vi "Beat_v2.vi"(7 "Name (\"\" to Use UUID)":string="Beat") -> ()   [LabVIEW 2025]
doc: "Compact code template for creating a CSM module without a user interface. The functionality of this template is identical to the CSM Module Template VI.\n\n\n> [!NOTE] <b>CSM Naming Rules</b>\n>\n> - CSM module name must be unique. Otherwise, CSM enters a `Critical Error` state.\n> - If the input module name is an empty string (\"\"), the system uses a UUID as the module name. Such a module is marked as standalone mode and does not appear in the module list.\n> - Worker Mode Rule: If the input module name ends with `#`, a worker mode node will be instantiated. Multiple worker mode nodes can form a worker mode module.\n> - Chain of Responsibility Mode Rule: If the input module name ends with `$` followed by a number, a chain of responsibility mode node will be instantiated. Multiple chain of responsibility mode nodes can form a chain of responsibility mode module.\n> - System-Level Module Rule: If the input module name starts with `.`, the module is a system-level module. Under default settings, such modules are not listed by the CSM - List Modules VI and are suitable for instantiating modules that run in the background.\n> - Submodule Rule: `.` is also allowed in a module name to separate the module name into multiple parts. CSM does not have strict rules for submodules. The `.` in the module name only marks the logical relationship between different modules. From an execution perspective, they are considered independent modules. The only difference is that you can obtain a list of logical submodules via the CSM - List Submodules VI.\n\n\n-- <b>Controls</b> --\n- <b>Name (\"\" to use UUID)</b>: CSM module name. Refer to <b>CSM Naming Rules</b> for module naming rules."
uses:
  <userlib>/_NEVSTOP/Communicable State Machine(CSM)/AdvanceAPI/CSM - Revert Arguments-Safe String.vi
  <userlib>/_NEVSTOP/Communicable State Machine(CSM)/_Shared/Trim Single-line Text.vi
  <userlib>/_NEVSTOP/Communicable State Machine(CSM)/AdvanceAPI/CSM - Break Down Multiple States String.vi
  <userlib>/_NEVSTOP/Communicable State Machine(CSM)/AdvanceAPI/CSM - Compact Multiple States.vi
  <userlib>/_NEVSTOP/Communicable State Machine(CSM)/AdvanceAPI/CSM - Make String Arguments Safe.vi
  <userlib>/_NEVSTOP/Communicable State Machine(CSM)/AdvanceAPI/CSM - Keywords.vi
  <userlib>/_NEVSTOP/Communicable State Machine(CSM)/Communicable State Machine.lvlib
panel:
  in  "Array 2":i32[](array[numeric])
  out "BeatInterval":i32
  out "State History":string
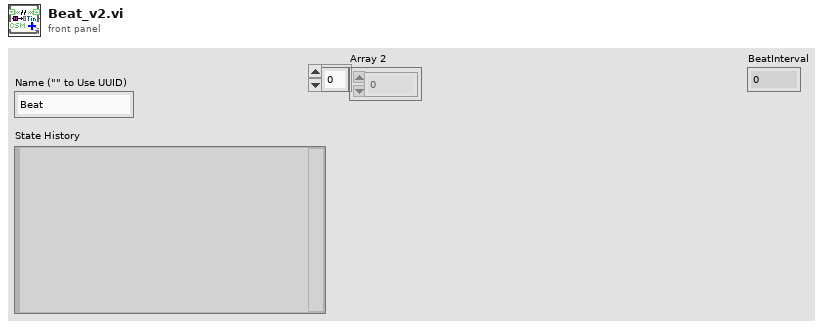
[diagram p1: front panel]
types:
  T1 = enum32{"Invalid", "Standard", "Closed", "Hidden", "Minimized", "Maximized"}
  T2 = enum32{"invalid app kind", "Development System", "Run Time System", "Student Edition", "Embedded LabVIEW", "Evaluation", "Custom"}
  T3 = typedef "Communicable State Machine.lvlib/_CSM_Response Source Message.ctl" = cluster{"‘State":string, "’Arguments":string, "’Error":errorcluster}
  T4 = cluster{"Current VI Reference":refnum<vi>, "Close Panel on Exit?":bool}
  T5 = cluster{"Core":cluster{"Current VI Reference":refnum<vi>, "Close Panel on Exit?":bool}, "BeatActive":bool, "T0":i32, "BeatInterval":i32, "N":i32}
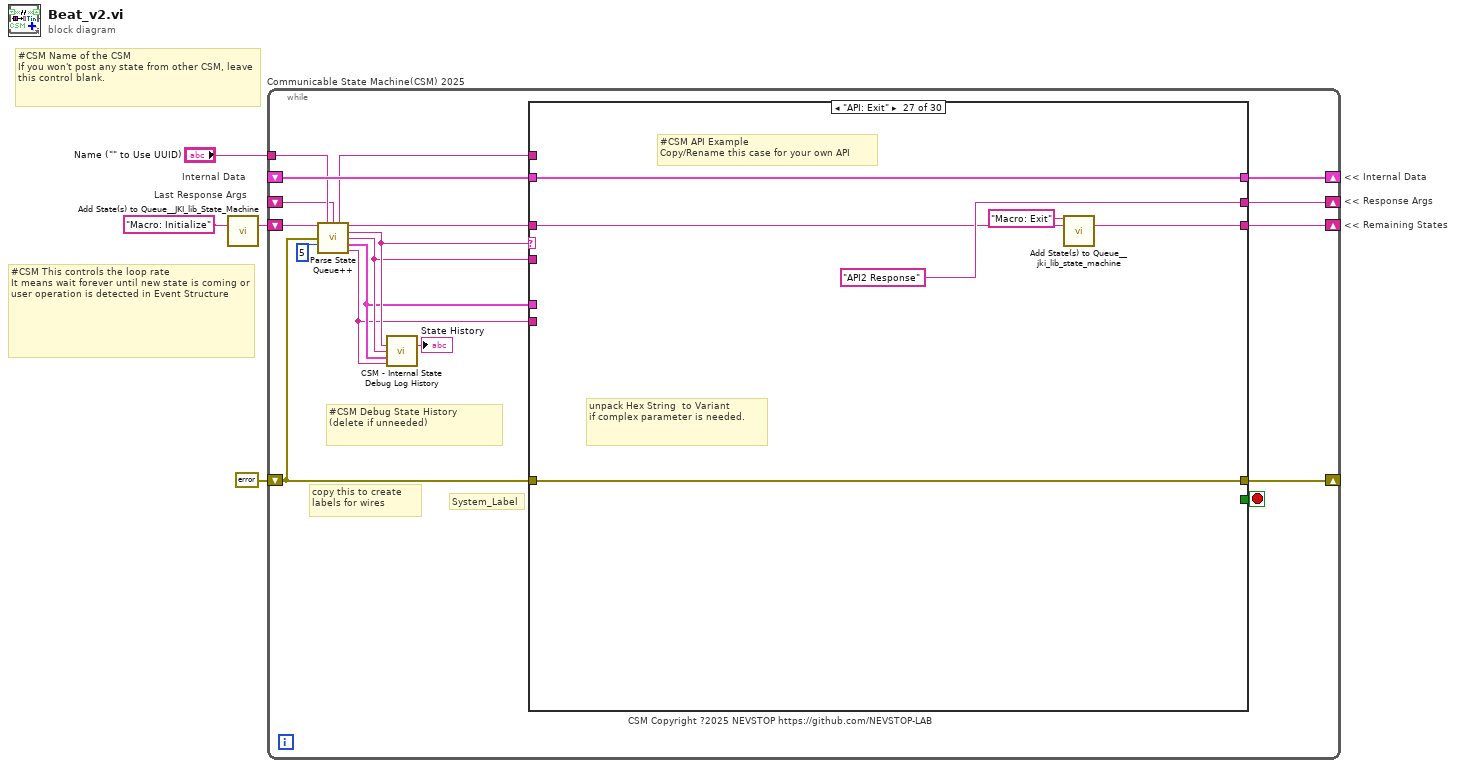
[diagram p0: block diagram]
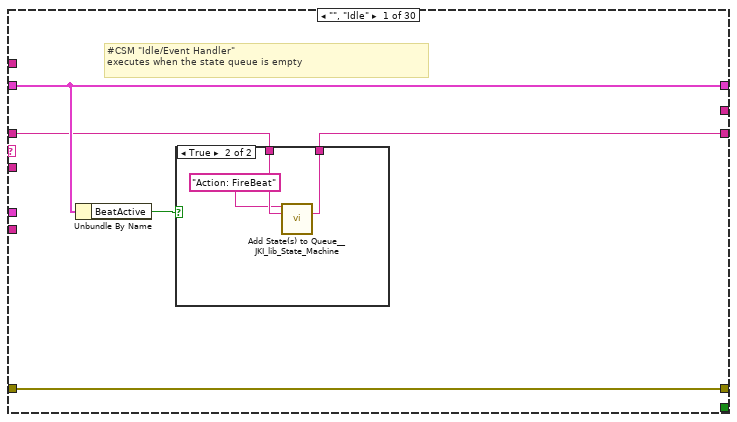
[diagram p2: hidden frame]
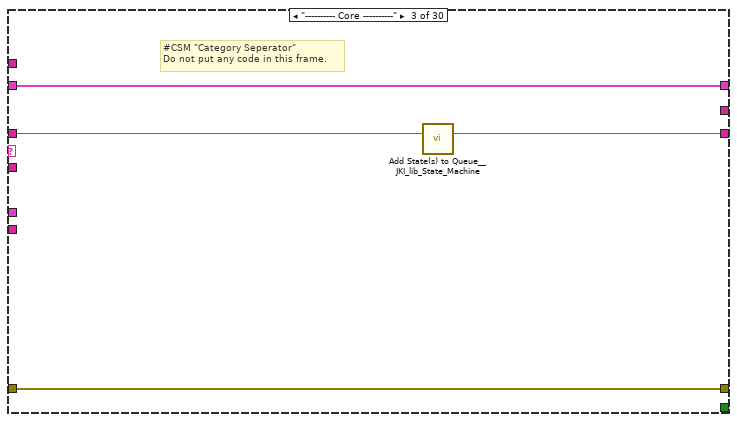
[diagram p5: hidden frame]
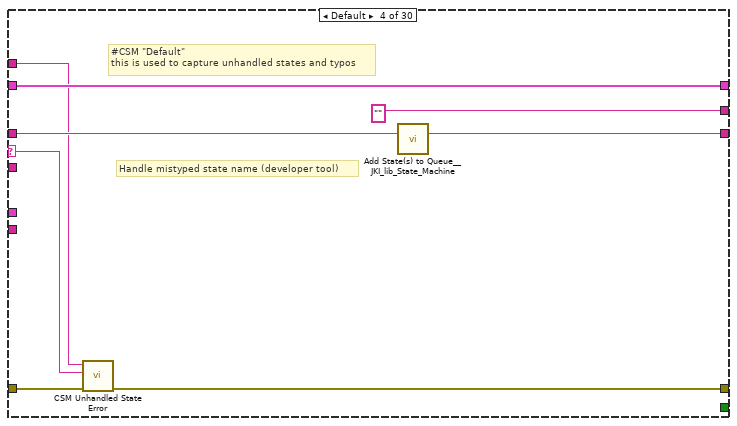
[diagram p6: hidden frame]
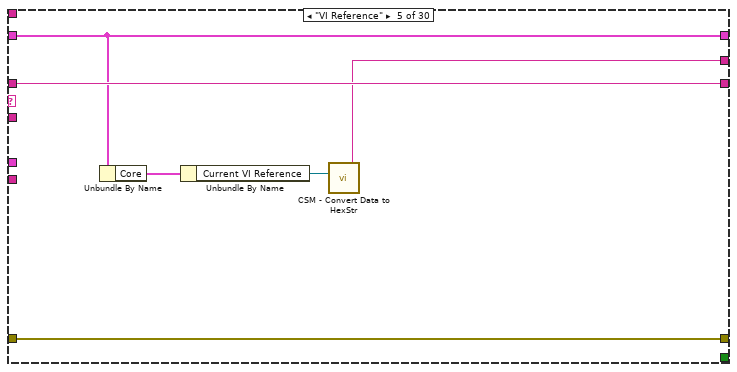
[diagram p7: hidden frame]
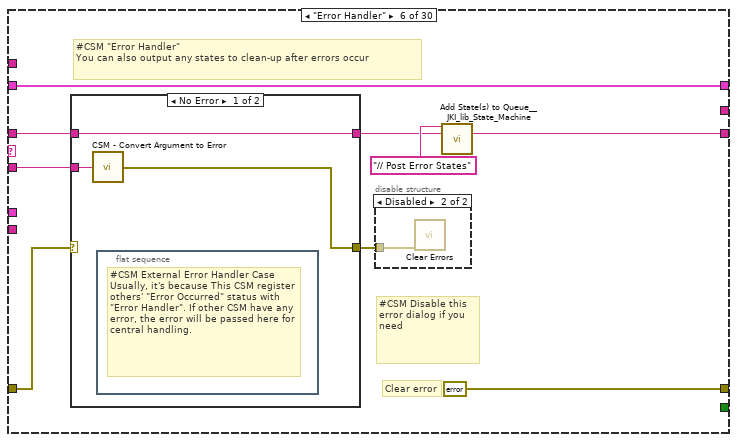
[diagram p8: hidden frame]
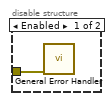
[diagram p9: hidden frame]
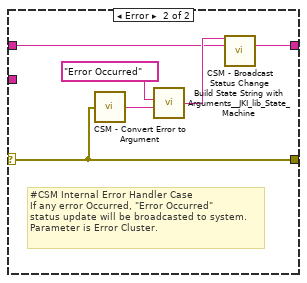
[diagram p10: hidden frame]
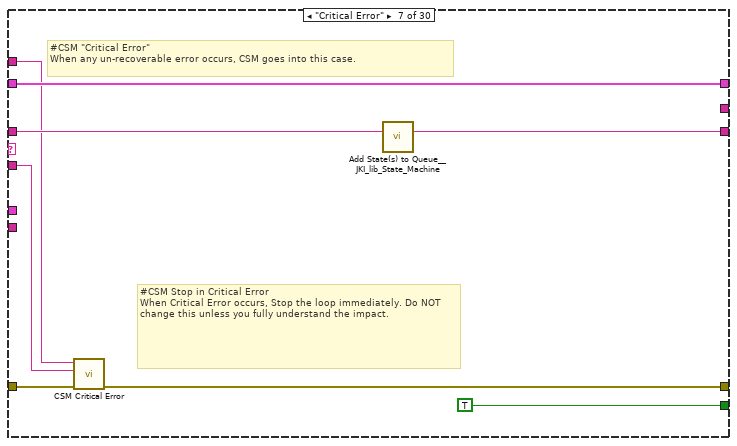
[diagram p11: hidden frame]
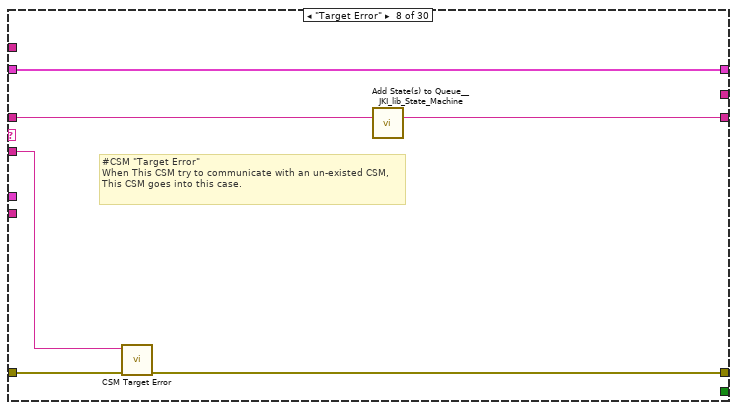
[diagram p12: hidden frame]
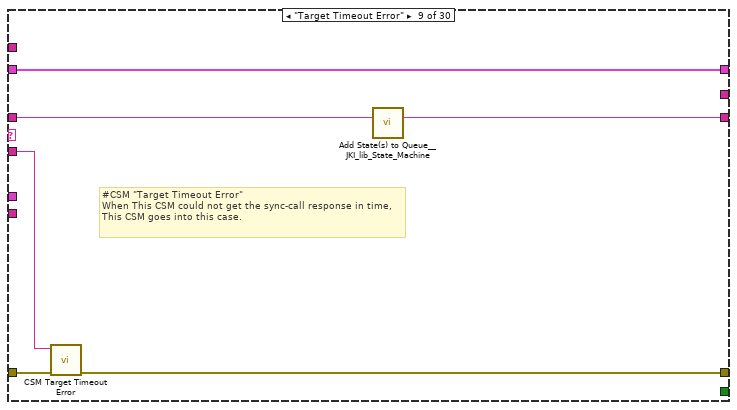
[diagram p13: hidden frame]
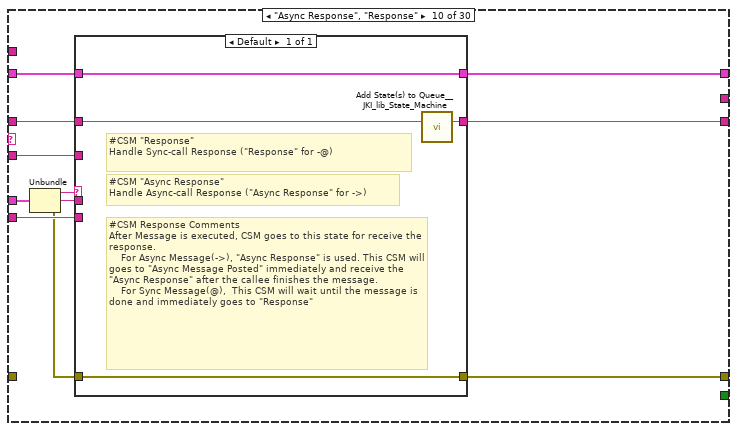
[diagram p14: hidden frame]
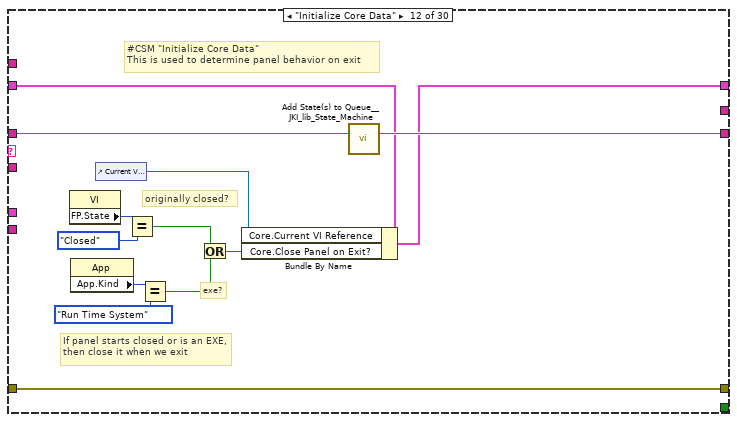
[diagram p16: hidden frame]
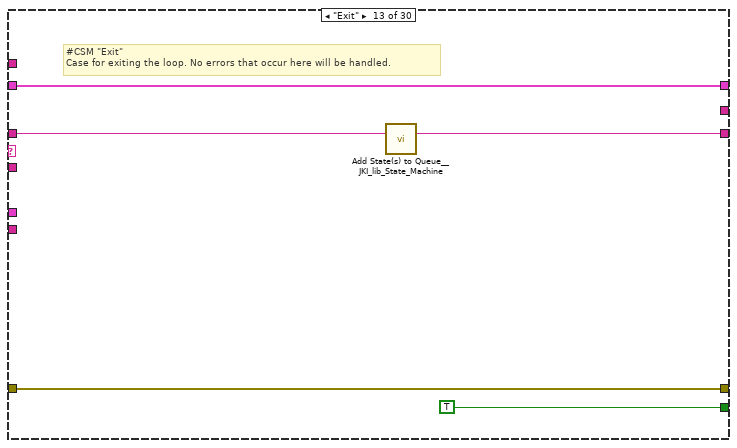
[diagram p17: hidden frame]
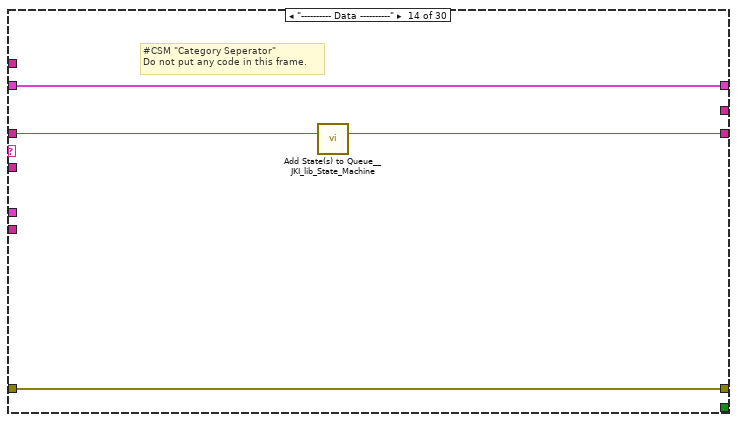
[diagram p18: hidden frame]
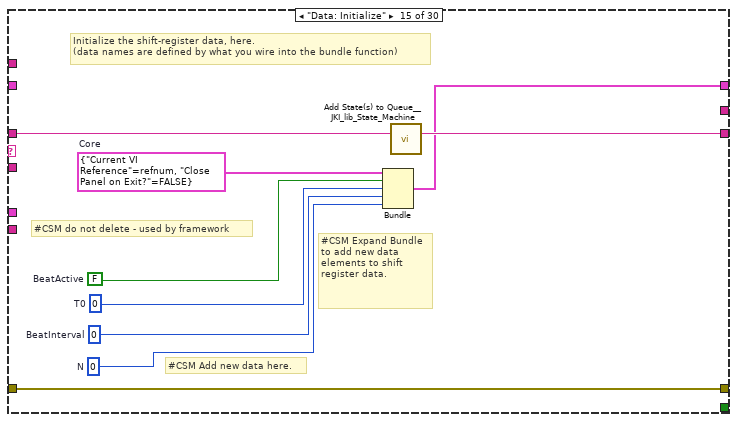
[diagram p19: hidden frame]
diagram:
  # "Last Response Args"
  # "Internal Data"
  # "#CSM Name of the CSM\nIf you won't post any state from other CSM, leave this control blank."
  # "#CSM This controls the loop rate\nIt means wait forever until new state is coming or user operation is detected in Event Structure"
  # "<< Internal Data"
  # "<< Response Args"
  # "<< Remaining States"
  n1 = call <vilib>:"Add State(s) to Queue__JKI_lib_State_Machine.vi"("State(s) in (\"\")"="Macro: Initialize" ("Init State(\"Macro: Initialize\")")) -> ("States Out"=w4:string)  [unwired: 14 in]
  n2 = while "Communicable State Machine(CSM) 2025" {
    shift-right: [w17] -> _
    shift-left: _ -> [w16]
    shift-right: [w20] -> _
    shift-left: errorcluster {"status"=FALSE, "code"=0, "source"=""} ("error out") -> [w15]
    shift-right: [w19] -> _
    shift-left: w4 -> [w21]
    tunnel: "Name (\"\" to Use UUID)" -> [w13]
    shift-right: [w14] -> _
    shift-left: _ -> [w7]
    stop <- w18 stop-if-true
    # "#CSM Debug State History\n(delete if unneeded)"
    # "copy this to create labels for wires"
    # "System_Label"
    # "CSM Copyright ?2025 NEVSTOP https://github.com/NEVSTOP-LAB"
    n3 = call <userlib>:"Parse State Queue++.vi"("State Queue"=w21, "Name (\"\" to Use UUID)"=w13, "Response Arguments"=w7, "Previous Error"=w15, "Dequeue (1 ms)"=5 ("Timeout")) -> ("Name Used"=w8:string, "Remaining States"=w22:string, "Current State"=w12:string, "Arguments"=w11:string, "Additional Information"=w10:T3, "Source CSM"=w9:string)  [unwired: 5 in]
    n4 = call <userlib>:"CSM - Internal State Debug Log History.vi"("State"=w12, "Arguments (\"\")"=w11, ">> Response Source Message >>"=w10, "Source (\"\")"=w9) -> ("Debug Log"=→"State History":string)  [unwired: 11 in]
    n5 = case shown="\"API: Exit\"" w12 {
      selector: w12 -> [_ _ _ w41 _ _ _ _ _ _ _ _ _ _ _ _ _ _ _ _ _ _ _ _ _ _ _ _ _ _]
      tunnel: w22 -> [w24 w33 w38 w45 w51 w57 w78 w84 w90 w98 w109 w123 w128 w132 w141 w143 w150 w154 w158 w164 w179 w248 w253 w260 w262 w266 w283 w291 w305 w321]
      tunnel: w11 -> [_ _ _ _ _ w56 w74 w83 w88 w97 _ _ _ _ _ _ _ _ _ w159 w173 _ _ _ _ w270 _ _ _ _]
      tunnel: w16 -> [w26 w32 w35 w43 w50 w60 w79 w85 w91 w100 w108 w116 w126 w129 _ w142 w145 w151 w156 w162 w175 w245 w250 w257 w261 w269 w286 w288 w292 w317]
      tunnel: [w27 w34 w36 w39 w52 errorcluster {"status"=FALSE, "code"=0, "source"=""} ("error out") w75 w81 w87 w103 w110 w120 w125 w130 w138 w144 w146 w152 w155 w160 w176 w246 w251 w258 w263 w281 w287 w289 w303 w319] -> w20
      tunnel: w15 -> [w27 w34 w36 w46 w52 w58 w80 w82 w89 _ w110 w120 w125 w130 w138 w144 w147 w152 w155 w161 w177 w246 w251 w258 w263 w281 w287 w289 w303 w319]
      tunnel: [w23 w33 w37 w44 w51 w53 w77 w86 w92 w99 w109 w122 w127 w131 w140 w143 w149 w153 w157 w163 w178 w247 w252 w259 w262 w267 w284 w290 w304 w320] -> w19
      tunnel: [_ _ _ _ _ _ TRUE _ _ _ _ _ TRUE _ _ _ _ _ _ _ _ _ _ _ _ _ _ _ _ _] -> w18
      tunnel: [w26 w32 w35 w43 w50 w60 w79 w85 w91 w101 w108 w121 w126 w129 w139 w142 w145 w151 w156 w162 w175 w245 w250 w257 w261 w268 w286 w288 w293 w318] -> w17
      tunnel: w9 -> [_ _ _ _ _ _ _ _ _ w95 _ _ _ _ _ _ _ _ _ _ _ _ _ _ _ _ _ _ _ _]
      tunnel: w10 -> [_ _ _ _ _ _ _ _ _ w102 _ _ _ _ _ _ _ _ _ _ _ _ _ _ _ _ _ _ _ _]
      tunnel: [_ _ _ "" w47 _ _ _ _ _ _ _ _ _ _ _ _ _ _ _ _ _ _ _ _ "API1 Response" "API2 Response" _ _ _] -> w14
      tunnel: w8 -> [_ _ _ w40 _ _ w73 _ _ _ _ _ _ _ _ _ _ _ _ _ _ _ _ _ _ _ _ _ _ _]
      frame "", "Idle" {
        # "#CSM \"Idle/Event Handler\"\nexecutes when the state queue is empty"
        n6 = Unbundle By Name(w26) -> ("BeatActive"=w25:bool)
        n7 = case shown="True" w25 {
          tunnel: w24 -> [w28 w31]
          tunnel: [w28 w30] -> w23
          frame False {
          }
          frame True {
            n8 = call <vilib>:"Add State(s) to Queue__JKI_lib_State_Machine.vi"("State(s) in Front (\"\")"="Action: FireBeat" ("State(s) in Front (\"\")"), "State(s) in (\"\")"=w31) -> ("States Out"=w30:string)  [unwired: 13 in]
          }
        }
      }
      frame "CSM Documentation" {
        # "#CSM README FIRST\n\nCommunicable State Machine(CSM) is a LabVIEW application framework that builds upon JKI State Machine(JKISM). It follows the pattern of JKISM and extends the keywords to describe message communication between modules, including concepts such as Sync-Message, Async-Message, Subscription/Unsubscription of status - essential elements for creating reusable code modules. For more information, please visit the CSM wiki: https://nevstop-lab.github.io/CSM-Wiki/\n\nFor instructions on JKI State Machine, visit: http://jki.net/state-machine/\nFor information about CSM, visit: https://github.com/NEVSTOP-LAB"
        # "#CSM \"Documentation\"\nCase for holding CSM Documenation"
      }
      frame "---------- Core ----------" {
        # "#CSM \"Category Seperator\"\nDo not put any code in this frame."
        n9 = call <vilib>:"Add State(s) to Queue__JKI_lib_State_Machine.vi"("State(s) in (\"\")"=w38) -> ("States Out"=w37:string)  [unwired: 14 in]
      }
      frame Default {
        # "#CSM \"Default\"\nthis is used to capture unhandled states and typos"
        # "Handle mistyped state name (developer tool)"
        n10 = call <userlib>:"CSM Unhandled State Error.vi"("error in (no error)"=w46, "Undefined State"=w41, "CSM Name"=w40) -> ("error out"=w39:errorcluster)  [unwired: 8 in]
        n11 = call <vilib>:"Add State(s) to Queue__JKI_lib_State_Machine.vi"("State(s) in (\"\")"=w45) -> ("States Out"=w44:string)  [unwired: 14 in]
      }
      frame "VI Reference" {
        n12 = Unbundle By Name(w50) -> ("Core"=w49:T4)
        n13 = Unbundle By Name(w49) -> ("Current VI Reference"=w48:refnum<vi>)
        n14 = call <userlib>:"CSM - Convert Data to HexStr.vi"("Variant"=w48) -> ("HEX String (0-9,A-F)"=w47:string)  [unwired: 8 in]
      }
      frame "Error Handler" {
        # "#CSM Disable this error dialog if you need"
        # "#CSM \"Error Handler\"\nYou can also output any states to clean-up after errors occur"
        # "Clear error"
        n15 = case shown="No Error" w58 {
          selector: w58 -> [_ w67]
          tunnel: [w66 w69] -> w54
          tunnel: w57 -> [w66 w68]
          tunnel: w56 -> [w65 _]
          tunnel: [w64 w67] -> w59
          frame No Error {
            n16 = call <userlib>:"CSM - Convert Argument to Error.vi"("Argument"=w65) -> ("Error"=w64:errorcluster)  [unwired: 4 in]
            n17 = flat-sequence {
              frame #0 {
                # "#CSM External Error Handler Case\nUsually, it's because This CSM register others' \"Error Occurred\" status with \"Error Handler\". If other CSM have any error, the error will be passed here for central handling."
              }
            }
          }
          frame Error {
            # "#CSM Internal Error Handler Case \nIf any error Occurred, \"Error Occurred\" \nstatus update will be broadcasted to system.\nParameter is Error Cluster."
            n18 = call <userlib>:"CSM - Convert Error to Argument.vi"("Error"=w67) -> ("Argument"=w71:string)  [unwired: 4 in]
            n19 = call <vilib>:"Build State String with Arguments__JKI_lib_State_Machine.vi"("Arguments (\"\")"=w71, "State"="Error Occurred" ("Status with Arguments")) -> ("State with Arguments"=w70:string)  [unwired: 4 in]
            n20 = call <userlib>:"CSM - Broadcast Status Change.vi"("Status With Arguments"=w70, "State Queue"=w68) -> ("Remaining States"=w69:string)  [unwired: 13 in]
          }
        }
        n21 = disable-structure shown="Disabled" {
          disable-tunnel: w59 -> [w62 w63]
          frame Enabled {
            n22 = call <vilib>:"General Error Handler.vi"("error in (no error)"=w62) -> ()  [unwired: 10 in, 5 out]
          }
          frame Disabled {
            n23 = call <vilib>:"Clear Errors.vi"("error in (no error)"=w63) -> ()  [unwired: 5 in, 2 out]
          }
        }
        n24 = call <vilib>:"Add State(s) to Queue__JKI_lib_State_Machine.vi"("State(s) in Front (\"\")"="// Post Error States", "State(s) in (\"\")"=w54) -> ("States Out"=w53:string)  [unwired: 13 in]
      }
      frame "Critical Error" {
        # "#CSM Stop in Critical Error\nWhen Critical Error occurs, Stop the loop immediately. Do NOT change this unless you fully understand the impact."
        # "#CSM \"Critical Error\"\nWhen any un-recoverable error occurs, CSM goes into this case."
        n25 = call <userlib>:"CSM Critical Error.vi"("error in (no error)"=w80, "Arugments (As Reason)"=w74, "CSM Name"=w73) -> ("error out"=w75:errorcluster)  [unwired: 8 in]
        n26 = call <vilib>:"Add State(s) to Queue__JKI_lib_State_Machine.vi"("State(s) in (\"\")"=w78) -> ("States Out"=w77:string)  [unwired: 14 in]
      }
      frame "Target Error" {
        # "#CSM \"Target Error\"\nWhen This CSM try to communicate with an un-existed CSM, This CSM goes into this case."
        n27 = call <userlib>:"CSM Target Error.vi"("error in (no error)"=w82, "Arguments (As CSM Name)"=w83) -> ("error out"=w81:errorcluster)  [unwired: 9 in]
        n28 = call <vilib>:"Add State(s) to Queue__JKI_lib_State_Machine.vi"("State(s) in (\"\")"=w84) -> ("States Out"=w86:string)  [unwired: 14 in]
      }
      frame "Target Timeout Error" {
        # "#CSM \"Target Timeout Error\"\nWhen This CSM could not get the sync-call response in time, This CSM goes into this case."
        n29 = call <userlib>:"CSM Target Timeout Error.vi"("error in (no error)"=w89, "Arguments (As CSM Name)"=w88) -> ("error out"=w87:errorcluster)  [unwired: 9 in]
        n30 = call <vilib>:"Add State(s) to Queue__JKI_lib_State_Machine.vi"("State(s) in (\"\")"=w90) -> ("States Out"=w92:string)  [unwired: 14 in]
      }
      frame "Async Response", "Response" {
        n31 = Unbundle(w102) -> ("‘State"=w96:string, "’Arguments"=w94:string, "’Error"=w93:errorcluster)
        n32 = case shown="Default" w96 {
          tunnel: [w107] -> w103
          tunnel: w93 -> [w107]
          tunnel: [w106] -> w101
          tunnel: w100 -> [w106]
          tunnel: [w104] -> w99
          tunnel: w98 -> [w105]
          tunnel: w97 -> [_]
          tunnel: w95 -> [_]
          tunnel: w94 -> [_]
          frame Default {
            # "#CSM Response Comments\nAfter Message is executed, CSM goes to this state for receive the response.\n    For Async Message(->), \"Async Response\" is used. This CSM will goes to \"Async Message Posted\" immediately and receive the \"Async Response\" after the callee finishes the message.\n    For Sync Message(@),  This CSM will wait until the message is done and immediately goes to \"Response\""
            # "#CSM \"Async Response\"\nHandle Async-call Response (\"Async Response\" for ->)"
            # "#CSM \"Response\"\nHandle Sync-call Response (\"Response\" for -@)"
            n33 = call <vilib>:"Add State(s) to Queue__JKI_lib_State_Machine.vi"("State(s) in (\"\")"=w105) -> ("States Out"=w104:string)  [unwired: 14 in]
          }
        }
      }
      frame "Async Message Posted" {
        # "#CSM \"Async Message Posted\"\nAfter Async Message is posted (-> or ->| ), CSM goes to this state for post-action.\nYou can use Argument - State to tell which Async Message is called."
      }
      frame "Initialize Core Data" {
        # "#CSM \"Initialize Core Data\"\nThis is used to determine panel behavior on exit"
        # "originally closed?"
        # "exe?"
        # "If panel starts closed or is an EXE, then close it when we exit"
        n34 = property class="VI"() -> ("FP.State"=w113:T1)  [unwired: 2 in, 2 out]
        n35 = property class="App"() -> ("App.Kind"=w119:T2)  [unwired: 2 in, 2 out]
        n36 = control-ref of="Current VI Reference"() -> (w114:refnum<vi>)
        n37 = Equal?(x=w113, y=T1."Closed" ("Front Panel Window:State")) -> (x = y?=w111:bool)
        n38 = Equal?(x=w119, y=T2."Run Time System" ("Application:Kind")) -> (x = y?=w117:bool)
        n39 = Or(x=w111, y=w117) -> (x .or. y?=w115:bool)
        n40 = Bundle By Name(cluster=w116, "Core.Current VI Reference"=w114, "Core.Close Panel on Exit?"=w115) -> (w121:T5)
        n41 = call <vilib>:"Add State(s) to Queue__JKI_lib_State_Machine.vi"("State(s) in (\"\")"=w123) -> ("States Out"=w122:string)  [unwired: 14 in]
      }
      frame "Exit" {
        # "#CSM \"Exit\"\nCase for exiting the loop. No errors that occur here will be handled."
        n42 = call <vilib>:"Add State(s) to Queue__JKI_lib_State_Machine.vi"("State(s) in (\"\")"=w128) -> ("States Out"=w127:string)  [unwired: 14 in]
      }
      frame "---------- Data ----------" {
        # "#CSM \"Category Seperator\"\nDo not put any code in this frame."
        n43 = call <vilib>:"Add State(s) to Queue__JKI_lib_State_Machine.vi"("State(s) in (\"\")"=w132) -> ("States Out"=w131:string)  [unwired: 14 in]
      }
      frame "Data: Initialize" {
        w133 = 0  # N
        w134 = 0  # BeatInterval
        w135 = 0  # T0
        w136 = FALSE  # BeatActive
        w137 = T4 {"Current VI Reference"=refnum, "Close Panel on Exit?"=FALSE}  # Core
        # "#CSM do not delete - used by framework"
        # "#CSM Expand Bundle to add new data elements to shift register data."
        # "#CSM Add new data here."
        # "Initialize the shift-register data, here.\n(data names are defined by what you wire into the bundle function)"
        n44 = Bundle("Core"=w137, "BeatActive"=w136, "T0"=w135, "BeatInterval"=w134, "N"=w133) -> (w139:T5)  [unwired: 1 in]
        n45 = call <vilib>:"Add State(s) to Queue__JKI_lib_State_Machine.vi"("State(s) in (\"\")"=w141) -> ("States Out"=w140:string)  [unwired: 14 in]
      }
      frame "Data: Update Indicators" {
      }
      frame "Data: Cleanup" {
        # "Cleanup any data and references, here.\n(this is called automatically, by the Macro: Exit)"
        n46 = Unbundle By Name(w145) -> ("Core.Current VI Reference"=w148:refnum<vi>)
        n47 = Close Reference(reference=w148, error in (no error)=w147) -> (error out=w146:errorcluster)
        n48 = call <vilib>:"Add State(s) to Queue__JKI_lib_State_Machine.vi"("State(s) in (\"\")"=w150) -> ("States Out"=w149:string)  [unwired: 14 in]
      }
      frame "---------- UI ----------" {
        # "#CSM \"Category Seperator\"\nDo not put any code in this frame."
        n49 = call <vilib>:"Add State(s) to Queue__JKI_lib_State_Machine.vi"("State(s) in (\"\")"=w154) -> ("States Out"=w153:string)  [unwired: 14 in]
      }
      frame "UI: Initialize" {
        # "#CSM \"UI: Initialize\"\nInitialize the User Interface, here.\n(this is called automatically, by the Macro: Init)"
        n50 = call <vilib>:"Add State(s) to Queue__JKI_lib_State_Machine.vi"("State(s) in (\"\")"=w158) -> ("States Out"=w157:string)  [unwired: 14 in]
      }
      frame "UI: Cursor Set" {
        # "#CSM \"UI: Cursor Set\"\nSet and Unset Cursor Busy.\n(Usage: \"UI: Cursor Set >> Busy|Idle\")"
        # "Argument"
        n51 = disable-structure shown="TARGET_TYPE!=Windows" {
          disable-tunnel: w161 -> [w167 w172]
          disable-tunnel: [w166 w172] -> w160
          disable-tunnel: w159 -> [w165 _]
          frame condition #0 (active) {
            n52 = case shown="\"Idle\", Default" w165 {
              tunnel: w167 -> [w169 w171]
              tunnel: [w168 w170] -> w166
              frame "Idle", Default {
                n53 = call <vilib>:"Unset Busy.vi"("error in (no error)"=w169) -> ("error out"=w168:errorcluster)  [unwired: 10 in]
              }
              frame "Busy" {
                n54 = call <vilib>:"Set Busy.vi"("error in (no error)"=w171) -> ("error out"=w170:errorcluster)  [unwired: 9 in, 1 out]
              }
            }
          }
          frame condition #1 {
          }
        }
        n55 = call <vilib>:"Add State(s) to Queue__JKI_lib_State_Machine.vi"("State(s) in (\"\")"=w164) -> ("States Out"=w163:string)  [unwired: 14 in]
      }
      frame "UI: Front Panel State" {
        # "#CSM \"UI: Front Panel State\"\nSet Front Panel Open or Closed\n(Usage: \"UI: Front Panel State >> Open|Close\")"
        # "Argument"
        n56 = Unbundle By Name(w175) -> ("Core.Current VI Reference"=w174:refnum<vi>)
        n57 = call <vilib>:"Add State(s) to Queue__JKI_lib_State_Machine.vi"("State(s) in (\"\")"=w179) -> ("States Out"=w178:string)  [unwired: 14 in]
        n58 = case shown="\"Close\", \"Closed\"" w173 {
          tunnel: w177 -> [w185 w200 w211 w224 w237]
          tunnel: [w187 w201 w213 w226 w239] -> w176
          tunnel: w174 -> [w186 w198 w212 w225 w238]
          frame "Open", "Standard", Default {
            w180 = T1."Standard" ("State")
            n59 = property class="VI"(reference=w186, error in=w185) -> (reference out=w183:refnum<vi>, error out=w184:errorcluster, "FP.State"=w182:T1)
            n60 = Not Equal?(x=w182, y=w180) -> (x != y?=w181:bool)
            n61 = case shown="True" w181 {
              tunnel: [w191 w193] -> w187
              tunnel: w184 -> [w190 w193]
              tunnel: w183 -> [w189 _]
              tunnel: w180 -> [w188 _]
              frame True {
                n62 = invoke class="VI" method="FP.Open"(reference=w189, error in=w190, "Activate"=TRUE, "State"=w188) -> (error out=w191:errorcluster)  [unwired: 1 in, 4 out]
              }
              frame False {
              }
            }
          }
          frame "Close", "Closed" {
            n63 = property class="VI"(reference=w198, error in=w200) -> (reference out=w197:refnum<vi>, error out=w199:errorcluster, "FP.State"=w195:T1)
            n64 = Not Equal?(x=w195, y=T1."Closed" ("Front Panel Window:State")) -> (x != y?=w194:bool)
            n65 = case shown="False" w194 {
              tunnel: [w202 w205] -> w201
              tunnel: w199 -> [w202 w204]
              tunnel: w197 -> [_ w203]
              frame False {
              }
              frame True {
                n66 = invoke class="VI" method="FP.Close"(reference=w203, error in=w204) -> (error out=w205:errorcluster)  [unwired: 1 in, 2 out]
              }
            }
          }
          frame "Hidden", "Hide" {
            w206 = T1."Hidden" ("State")
            n67 = property class="VI"(reference=w212, error in=w211) -> (reference out=w209:refnum<vi>, error out=w210:errorcluster, "FP.State"=w208:T1)
            n68 = Not Equal?(x=w208, y=w206) -> (x != y?=w207:bool)
            n69 = case shown="True" w207 {
              tunnel: [w217 w218] -> w213
              tunnel: w210 -> [w216 w218]
              tunnel: w209 -> [w215 _]
              tunnel: w206 -> [w214 _]
              frame True {
                n70 = invoke class="VI" method="FP.Open"(reference=w215, error in=w216, "State"=w214) -> (error out=w217:errorcluster)  [unwired: 2 in, 4 out]
              }
              frame False {
              }
            }
          }
          frame "Minimize", "Minimized" {
            w219 = T1."Minimized" ("State")
            n71 = property class="VI"(reference=w225, error in=w224) -> (reference out=w222:refnum<vi>, error out=w223:errorcluster, "FP.State"=w221:T1)
            n72 = Not Equal?(x=w221, y=w219) -> (x != y?=w220:bool)
            n73 = case shown="True" w220 {
              tunnel: [w230 w231] -> w226
              tunnel: w223 -> [w229 w231]
              tunnel: w222 -> [w228 _]
              tunnel: w219 -> [w227 _]
              frame True {
                n74 = invoke class="VI" method="FP.Open"(reference=w228, error in=w229, "State"=w227) -> (error out=w230:errorcluster)  [unwired: 2 in, 4 out]
              }
              frame False {
              }
            }
          }
          frame "Maximize", "Maximized" {
            w232 = T1."Maximized" ("State")
            n75 = property class="VI"(reference=w238, error in=w237) -> (reference out=w235:refnum<vi>, error out=w236:errorcluster, "FP.State"=w234:T1)
            n76 = Not Equal?(x=w234, y=w232) -> (x != y?=w233:bool)
            n77 = case shown="True" w233 {
              tunnel: [w243 w244] -> w239
              tunnel: w236 -> [w242 w244]
              tunnel: w235 -> [w241 _]
              tunnel: w232 -> [w240 _]
              frame True {
                n78 = invoke class="VI" method="FP.Open"(reference=w241, error in=w242, "State"=w240) -> (error out=w243:errorcluster)  [unwired: 2 in, 4 out]
              }
              frame False {
              }
            }
          }
        }
      }
      frame "---------- Macro ----------" {
        # "#CSM \"Category Seperator\"\nDo not put any code in this frame."
        n79 = call <vilib>:"Add State(s) to Queue__JKI_lib_State_Machine.vi"("State(s) in (\"\")"=w248) -> ("States Out"=w247:string)  [unwired: 14 in]
      }
      frame "Macro: Initialize" {
        # "#CSM \"Macro: Initialize\"\nInitialization Macro (This is called once, when the VI starts)"
        n80 = call <vilib>:"Add State(s) to Queue__JKI_lib_State_Machine.vi"("State(s) in Front (\"\")"="Data: Initialize\nInitialize Core Data\nData: Update Indicators", "State(s) in (\"\")"=w253) -> ("States Out"=w252:string)  [unwired: 13 in]
      }
      frame "Macro: Exit" {
        # "#CSM \"Macro: Exit\"\nExit Macro (This is called once, when the VI exits)"
        n81 = call <vilib>:"Add State(s) to Queue__JKI_lib_State_Machine.vi"("State(s) in Front (\"\")"="//Exit Sub-Modules ", "State(s) at Back (\"\")"="Data: Cleanup\nExit") -> ("States Out"=w255:string)  [unwired: 13 in]
        n82 = call <vilib>:"Add State(s) to Queue__JKI_lib_State_Machine.vi"("State(s) in Front (\"\")"=w255, "State(s) in (\"\")"=w260) -> ("States Out"=w259:string)  [unwired: 13 in]
      }
      frame "---------- API ----------" {
        # "#CSM \"Category Seperator\"\nDo not put any code in this frame."
      }
      frame "API: StartBeat" {
        # "Reset NoteIndex\nand set BeatActive"
        # "Get T0 and BeatInterval by setting up\n element index as 0 and 1"
        # "#CSM API Example\nCopy/Rename this case for your own API"
        # "#CSM >> Msg/Rep's CSM >>\nIf you need to tell who triggered this state , use this string. If it's this case itself, this string is \"\"."
        # "#CSM >> Arguments >>\nDeal with the parameter if any"
        n83 = Spreadsheet String To Array(delimiter (Tab)=",", format string="%d", spreadsheet string=w270, array type (2D Dbl)="Array 2") -> (array=w277:i32[])
        n84 = Index Array(array=w277, index #1=0 ("index"), index #2=1 ("index")) -> (element #1=w274:i32, element #2=w273:i32)
        n85 = Bundle By Name(cluster=w269, "T0"=w274, "BeatInterval"=w273, "N"=0 ("NoteIndex"), "BeatActive"=TRUE) -> (w268:T5)
        n86 = call <vilib>:"Add State(s) to Queue__JKI_lib_State_Machine.vi"("State(s) in Front (\"\")"="Action: FireBeat" ("State(s) in Front (\"\")"), "State(s) in (\"\")"=w266) -> ("States Out"=w267:string)  [unwired: 13 in]
      }
      frame "API: Exit" {
        # "#CSM API Example\nCopy/Rename this case for your own API"
        # "unpack Hex String  to Variant\nif complex parameter is needed."
        n87 = call <vilib>:"Add State(s) to Queue__jki_lib_state_machine.vi"("State(s) in Front (\"\")"="Macro: Exit" ("State(s) in Front (\"\")"), "State(s) in (\"\")"=w283) -> ("States Out"=w284:string)  [unwired: 13 in]
      }
      frame "---------- Action ----------" {
        # "#CSM \"Category Seperator\"\nDo not put any code in this frame."
        n88 = call <vilib>:"Add State(s) to Queue__JKI_lib_State_Machine.vi"("State(s) in (\"\")"=w291) -> ("States Out"=w290:string)  [unwired: 14 in]
      }
      frame "Action: FireBeat" {
        # "Index of the\n note array"
        # "When Current Time >= Expected Time\nIt is the time to beep"
        # "Current Time"
        # "Expected Time\nThe exact clock time the\nnext beep should happen"
        # "#CSM \"Internal State\"\nThis category is used for holding internal states"
        n89 = Unbundle By Name(w292) -> ("T0"=w302:i32, "BeatInterval"=w299:i32, "N"=w301:i32)
        "BeatInterval" <- w299
        n90 = Add(x=w301, y=1) -> (x+y=w298:i32)
        n91 = Multiply(x=w299, y=w298) -> (x*y=w297:i32)
        n92 = Add(x=w302, y=w297) -> (x+y=w295:i32)
        n93 = Tick Count (ms)() -> (millisecond timer value=w294:u32)
        n94 = Greater Or Equal?(x=w294, y=w295) -> (x >= y?=w296:bool)
        n95 = case shown="True" w296 {
          tunnel: w292 -> [w306 w312]
          tunnel: [w306 w311] -> w293
          tunnel: w292 -> [_ w307]
          frame False {
          }
          frame True {
            # "Index++"
            n96 = call <vilib>:"Beep.vi"("use system alert? (T)"=FALSE, "duration (msec)"=u32 150, "frequency (Hz)"=u32 1000) -> ()  [unwired: 9 in]
            n97 = Unbundle By Name(w307) -> ("N"=w309:i32)
            n98 = Add(x=w309, y=1.0) -> (x+y=w310:dbl)
            n99 = Bundle By Name(cluster=w312, "N"=w310) -> (w311:T5)
          }
        }
        n100 = call <vilib>:"Add State(s) to Queue__JKI_lib_State_Machine.vi"("State(s) in (\"\")"=w305) -> ("States Out"=w304:string)  [unwired: 14 in]
      }
      frame "API: StopBeat" {
        # "#CSM \"Internal State\"\nThis category is used for holding internal states"
        n101 = Bundle By Name(cluster=w317, "BeatActive"=FALSE) -> (w318:T5)
        n102 = call <vilib>:"Add State(s) to Queue__JKI_lib_State_Machine.vi"("State(s) in (\"\")"=w321) -> ("States Out"=w320:string)  [unwired: 14 in]
      }
    }
  }
